vi "s-1 rastgele üretilen 15 sayıyı 15 ile çarpıp 5 çıkartıp tam sayı yapan program 2018 19.vi"() -> ()   [LabVIEW 2014]
panel:
  out "aa":dbl
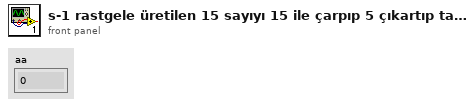
[diagram p1: front panel]
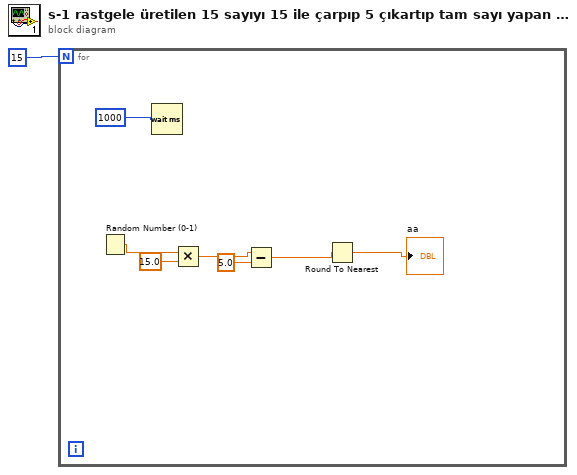
[diagram p0: block diagram]
diagram:
  n1 = for {
    N: 15 -> [_]
    n2 = Random Number (0-1)() -> (number: 0 to 1=w7:dbl)
    n3 = Wait (ms)(milliseconds to wait=u32 1000 ("millisecond timer value")) -> ()  [unwired: 1 out]
    n4 = Multiply(x=w7, y=15.0) -> (x*y=w5:dbl)
    n5 = Subtract(x=w5, y=5.0) -> (x-y=w3:dbl)
    n6 = Round To Nearest(number=w3) -> (nearest integer value=→"aa":dbl)
  }
